vi "计算数值.vi"(1 "表达式":string) -> (0 "结果":string)   [LabVIEW 2014]
panel:
  out "表达式 2":string
  out "替换子字符串":string
  out "子字符串":string
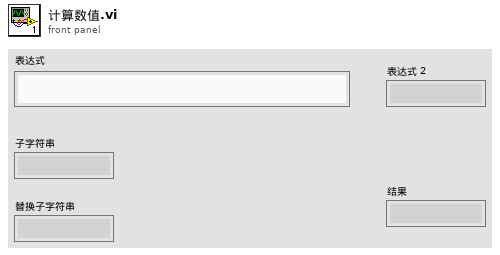
[diagram p1: front panel]
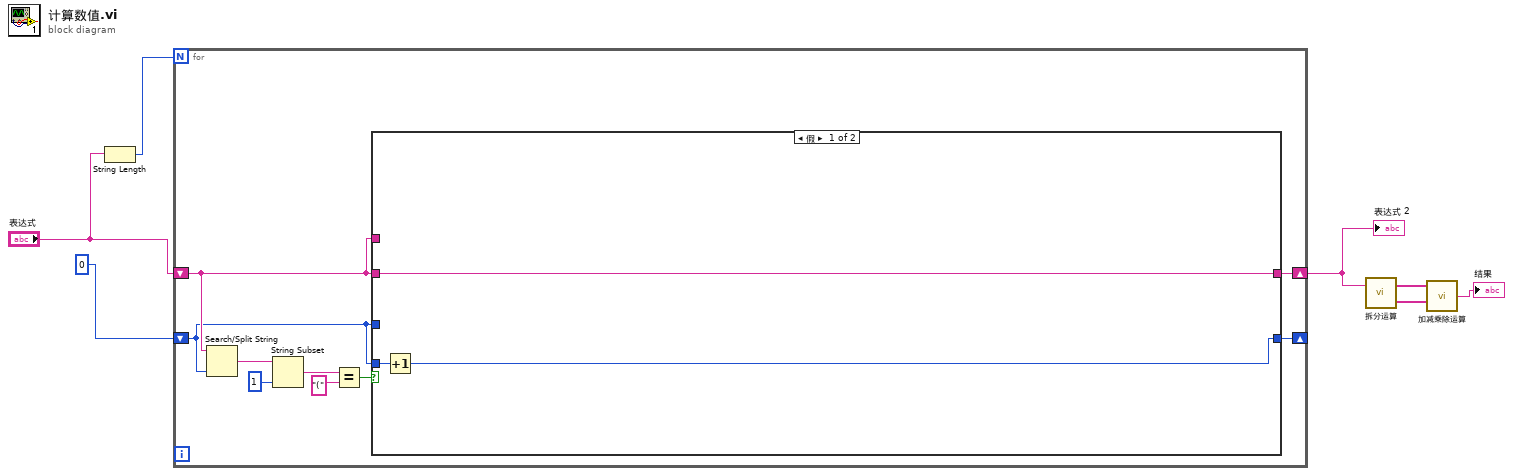
[diagram p0: block diagram]
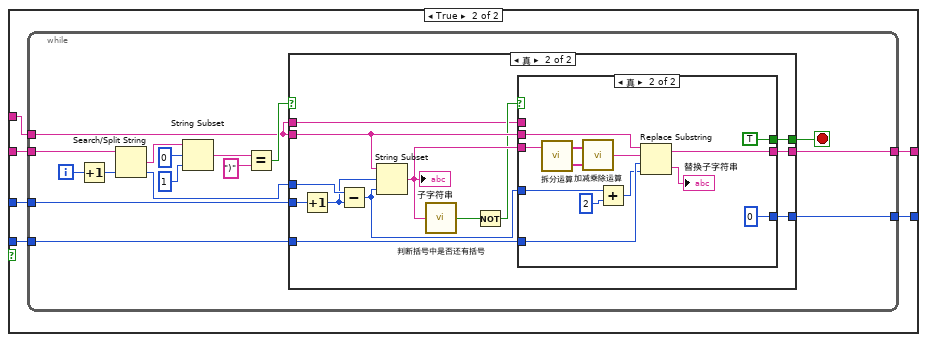
[diagram p2: hidden frame]
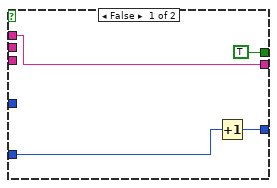
[diagram p4: hidden frame]
diagram:
  n1 = String Length(string="表达式") -> (length=w5:i32)
  n2 = for {
    N: w5 -> [_]
    shift-right: [w13] -> w4
    shift-left: "表达式" -> [w14]
    shift-right: [w12] -> _
    shift-left: 0 -> [w8]
    n3 = Search/Split String(string=w14, offset (0)=w8) -> (match + rest of string=w11:string)  [unwired: 1 in, 2 out]
    n4 = String Subset(string=w11, length (rest)=1 ("长度（剩余）")) -> (substring=w10:string)  [unwired: 1 in]
    n5 = Equal?(x=w10, y="(") -> (x = y?=w15:bool)
    n6 = case shown="假" w15 {
      tunnel: w14 -> [w17 w25]
      tunnel: w14 -> [_ w24]
      tunnel: w8 -> [_ w23]
      tunnel: w8 -> [w19 w22]
      tunnel: [w17 w21] -> w13
      tunnel: [w18 w20] -> w12
      frame False {
        n7 = Increment(x=w19) -> (x+1=w18:i32)
      }
      frame True {
        n8 = while {
          tunnel: w24 -> [w27]
          tunnel: w23 -> [w33]
          tunnel: w22 -> [w31]
          tunnel: [w30] -> w21
          tunnel: [w26] -> w20
          tunnel: w25 -> [w41]
          i -> [w40]
          stop <- w28 stop-if-true
          n9 = Increment(x=w40) -> (x+1=w39:i32)
          n10 = Search/Split String(string=w41, offset (0)=w39) -> (match + rest of string=w37:string, offset of match=w32:i32)  [unwired: 1 in, 1 out]
          n11 = String Subset(string=w37, offset (0)=0 ("偏移量(0)"), length (rest)=1 ("长度（剩余）")) -> (substring=w36:string)
          n12 = Equal?(x=w36, y=")") -> (x = y?=w29:bool)
          n13 = case shown="真" w29 {
            tunnel: w27 -> [_ w52]
            tunnel: w33 -> [_ w53]
            tunnel: w32 -> [_ w54]
            tunnel: w31 -> [_ w51]
            tunnel: [_ w50] -> w30
            tunnel: [_ w44] -> w28
            tunnel: w27 -> [_ w43]
            tunnel: [_ w42] -> w26
            frame False {
            }
            frame True {
              n14 = Increment(x=w53) -> (x+1=w49:i32)
              n15 = Subtract(x=w54, y=w49) -> (x-y=w48:i32)
              n16 = String Subset(string=w52, offset (0)=w49, length (rest)=w48) -> (substring=w47:string)
              "子字符串" <- w47
              n17 = call "判断括号中是否还有括号.vi"("字符串"=w47) -> ("布尔"=w46:bool)
              n18 = Not(x=w46) -> (.not. x?=w45:bool)
              n19 = case shown="真" w45 {
                tunnel: w47 -> [_ w61]
                tunnel: w52 -> [_ w71]
                tunnel: w51 -> [w57 w70]
                tunnel: [w58 w69] -> w50
                tunnel: w48 -> [_ w66]
                tunnel: [TRUE TRUE] -> w44
                tunnel: w43 -> [w58 _]
                tunnel: [w56 0] -> w42
                frame False {
                  n20 = Increment(x=w57) -> (x+1=w56:i32)
                }
                frame True {
                  n21 = call "拆分运算.vi"("公式"=w61) -> ("符号"=w59:string[], "元素"=w60:string[])  [unwired: 1 in]
                  n22 = call "加减乘除运算.vi"("符号"=w59, "元素"=w60) -> ("结果"=w68:string)
                  n23 = Add(x=w66, y=2) -> (x+y=w65:i32)
                  n24 = Replace Substring(2:w65, 3:w70, 4:w68, 5:w71) -> (0:→"替换子字符串":string, 1:w69:string)
                }
              }
            }
          }
        }
      }
    }
  }
  "表达式 2" <- w4
  n25 = call "拆分运算.vi"("公式"=w4) -> ("符号"=w2:string[], "元素"=w3:string[])  [unwired: 1 in]
  n26 = call "加减乘除运算.vi"("符号"=w2, "元素"=w3) -> ("结果"=→"结果":string)
